vi "SlashCodesAndStringConstants.vi"() -> ()   [LabVIEW 2019]
panel:
  out "concatenated string":string
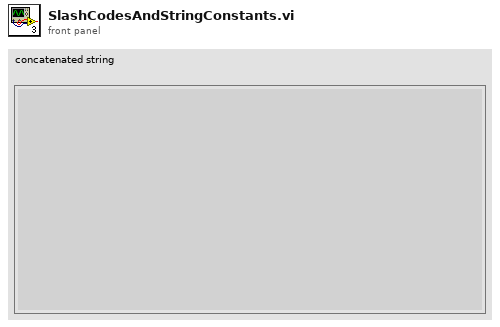
[diagram p1: front panel]
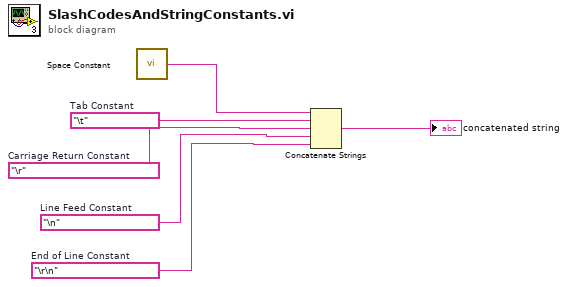
[diagram p0: block diagram]
diagram:
  w2 = "\r\n"  # End of Line Constant
  w3 = "\n"  # Line Feed Constant
  w4 = "\r"  # Carriage Return Constant
  w5 = "\t"  # Tab Constant
  n1 = call <vilib>:"Space Constant.vi"() -> ("String"=w6:string)
  n2 = Concatenate Strings(w6, w5, w4, w3, w2) -> (→"concatenated string":string)
